vi "Write GeneType.vi"(8 "error in (no error)":errorcluster, 10 "GeneType":T1, 11 "IGene in":refnum<class "IGene.lvclass">) -> (0 "error out":errorcluster, 3 "IGene out":refnum<class "IGene.lvclass">)   [LabVIEW 2016, in "IGene.lvclass"]
uses:
  IGene.lvclass
  _typedefs/IGene_GeneType.ctl
  IGene.lvclass/IGene.ctl
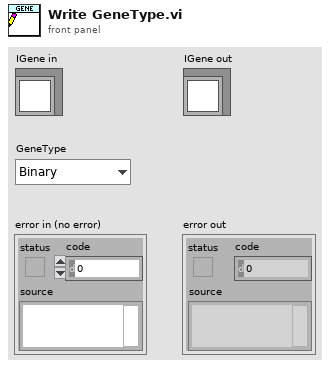
[diagram p1: front panel]
types:
  T1 = typedef "IGene.lvclass/IGene_GeneType.ctl" = enum16{"Binary", "Real", "Object", "None"}
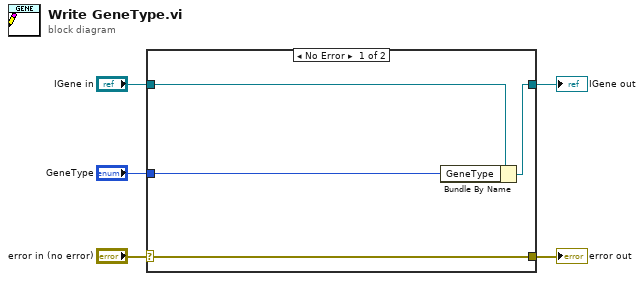
[diagram p0: block diagram]
diagram:
  n1 = case shown="No Error" "error in (no error)" {
    selector: "error in (no error)" -> [w9 w10]
    tunnel: [w9 w10] -> w4
    tunnel: [w7 w11] -> w2
    tunnel: "IGene in" -> [w8 w11]
    tunnel: "GeneType" -> [w6 _]
    frame No Error {
      n2 = Bundle By Name(cluster=w8, "GeneType"=w6) -> (w7:refnum<class "IGene.lvclass">)
    }
    frame Error {
    }
  }
  "error out" <- w4
  "IGene out" <- w2
